vi "comm flush.vi"(8 "error in (no error)":errorcluster, 10 "Flags (0x08)":u32=8 format="%.0x", 11 "Comm Handle":u32) -> (0 "error out":errorcluster, 3 "dup Comm Handle":u32)   [LabVIEW 2013, in "lvserial.lvlib"]
doc: "COMM_FLUSH_TXABORT 0x0001 \nTerminates all outstanding overlapped write operations and returns immediately, even if the write operations have not been completed.\n\nCOMM_FLUSH_RXABORT 0x0002 \nTerminates all outstanding overlapped read operations and returns immediately, even if the read operations have not been completed.\n\nCOMM_FLUSH_TXCLEAR 0x0004 \nClears the output buffer.\n\nCOMM_FLUSH_RXCLEAR 0x0008\nClears the input buffer."
uses:
  lvserial.lvlib
  lvserial.dll
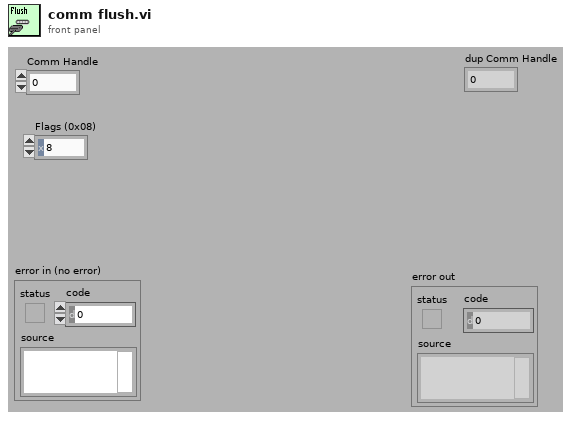
[diagram p1: front panel]
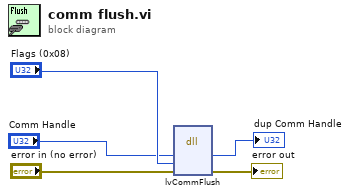
[diagram p0: block diagram]
diagram:
  n1 = dll-call lib="lvserial.dll" fn="lvCommFlush"("hComm"="Comm Handle", "ulFlags"="Flags (0x08)", "error in (no error)"="error in (no error)") -> ("hComm"=→"dup Comm Handle":u32, "error in (no error)"=→"error out":errorcluster)  [unwired: 4 in, 3 out]
